vi "人脸识别程序_调用DB匹配_模板匹配.vi"() -> (1 "识别结果":string, 2 "匹配图像":T1(plugin-control))   [LabVIEW 2017]
uses:
  <vilib>/vision/NI_Vision_Development_Module.lvlib
panel:
  out "匹配图像路径":path
  out "Score":sgl
  out "识别成功":bool
  out "添加的路径":path
  out "Number of Matches":i32
  out "Matches (pixel)":T2(array[cluster]) {"Bounding Box"."y" format="%.2f"; "Bounding Box"."x" format="%.2f"; "Score" format="%.2f"; "Scale" format="%.2f"; "Angle" format="%.2f"; "Position"."y" format="%.2f"; "Position"."x" format="%.2f"}
  out "模板图像":T1(plugin-control)
  in  "人脸DB基路径":path=path "D:/机器视觉_短学期/课程项目/人脸图像DB"
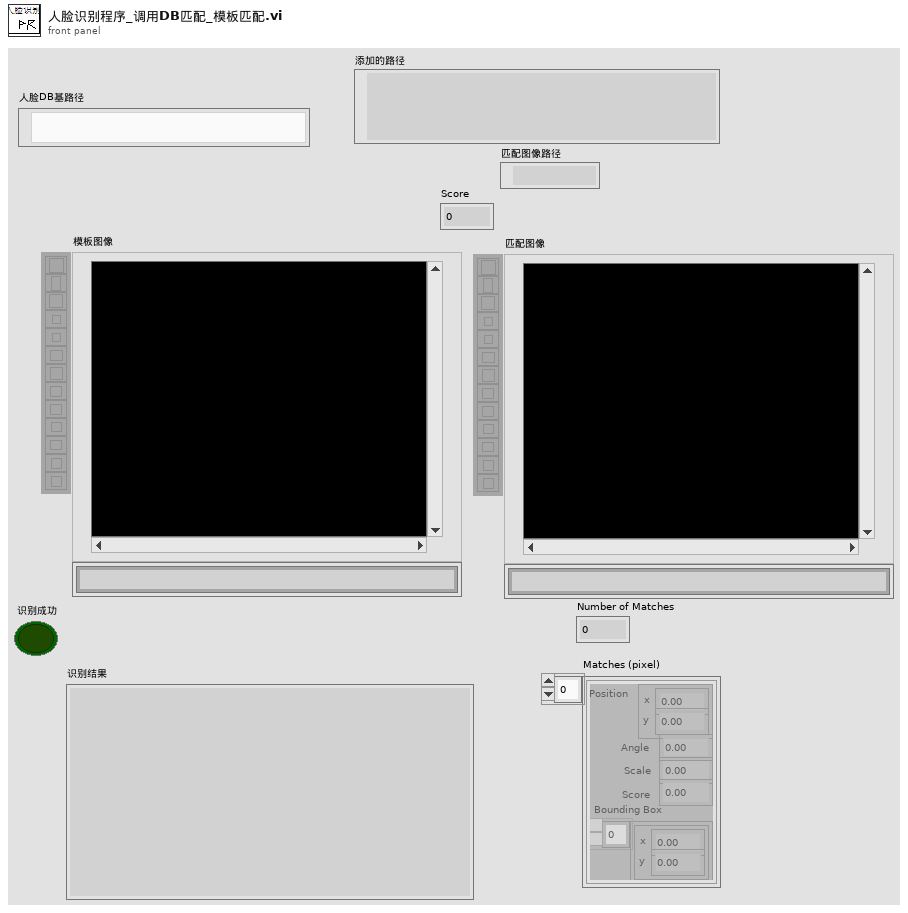
[diagram p1: front panel]
types:
  T1 = typedef "IMAQ Image.ctl" = refnum<image>
  T2 = cluster{"Position":cluster{"x":sgl, "y":sgl}, "Angle":sgl, "Scale":sgl, "Score":sgl, "Bounding Box":cluster{"x":sgl, "y":sgl}[]}[]
  T3 = typedef "Image Type" = u32
  T4 = cluster{"Position":cluster{"x":sgl, "y":sgl}, "Angle":sgl, "Scale":sgl, "Score":sgl, "Bounding Box":cluster{"x":sgl, "y":sgl}[]}
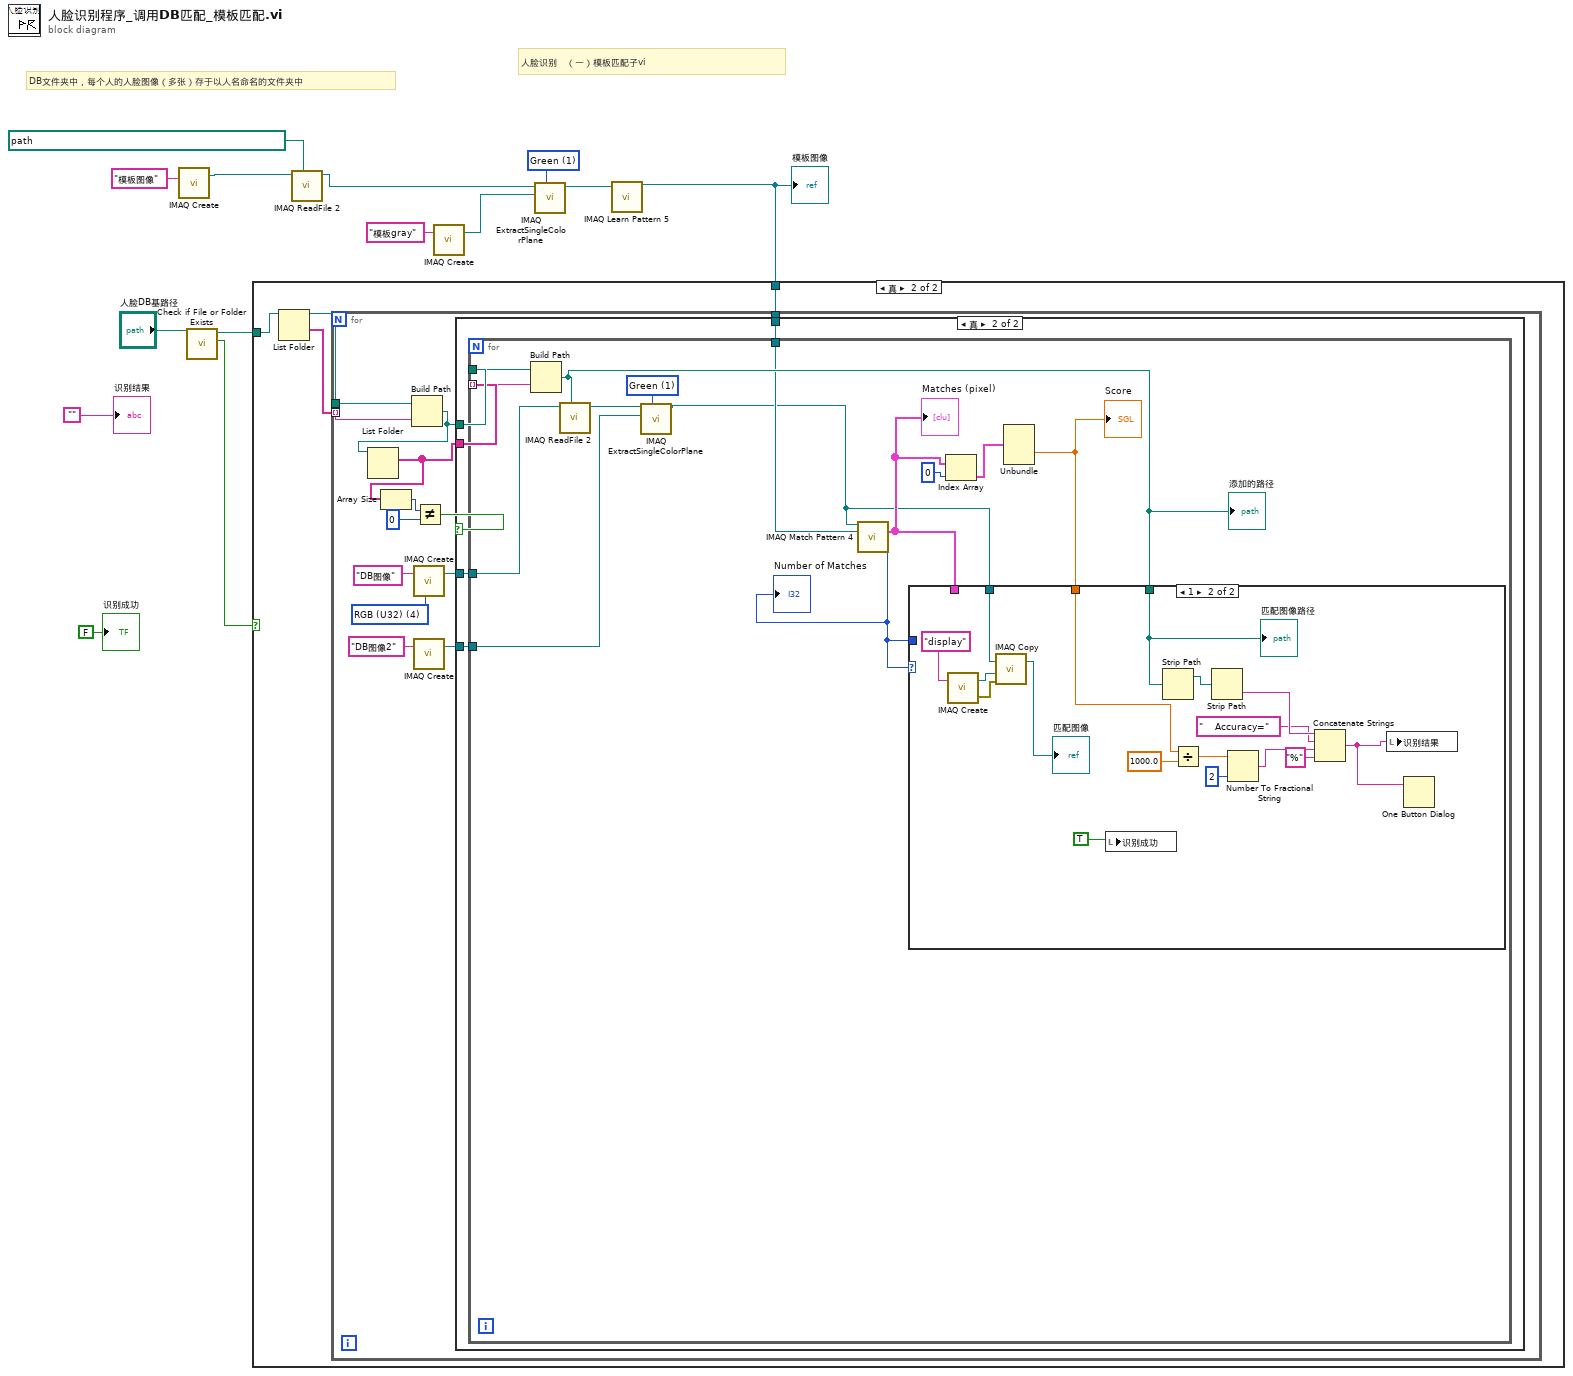
[diagram p0: block diagram]
diagram:
  w11 = 1 items=["Red", "Green", "Blue", "Hue", "Saturation", "Luminance", "Value", "Intensity"] ("Color Plane")
  # "人脸识别   （一）模板匹配子vi"
  # "DB文件夹中，每个人的人脸图像（多张）存于以人名命名的文件夹中"
  n1 = call "IMAQ Create"("Image Name"="模板图像") -> ("New Image"=w4:T1)  [unwired: 4 in, 1 out]
  n2 = call <vilib>:"Check if File or Folder Exists.vi"("path"="人脸DB基路径") -> ("file or folder exists?"=w13:bool, "dup path"=w12:path)  [unwired: 8 in, 1 out]
  n3 = call "IMAQ ReadFile 2"("File Path"=path "D:/机器视觉_短学期/课程项目/人脸图像DB/5.jpg", "Image"=w4) -> ("Image Out"=w1:T1)  [unwired: 5 in, 4 out]
  n4 = call "IMAQ Create"("Image Name"="模板gray") -> ("New Image"=w6:T1)  [unwired: 4 in, 1 out]
  n5 = call "IMAQ ExtractSingleColorPlane"("Color Plane"=w11, "Image Dst"=w6, "Image Src"=w1) -> ("Image Dst Out"=w10:T1)  [unwired: 7 in, 1 out]
  n6 = call "IMAQ Learn Pattern 5"("Image"=w10) -> ("Template Image Out"=w9:T1)  [unwired: 12 in, 2 out]
  "模板图像" <- w9
  n7 = case shown="真" w13 {
    tunnel: w12 -> [_ w18]
    tunnel: w9 -> [_ w15]
    frame False {
    }
    frame True {
      n8 = List Folder(path=w18) -> (path out=w17:path, folder names=w16:string[])  [unwired: 3 in, 2 out]
      n9 = for {
        tunnel: w16 -> [w31] mode=indexing
        tunnel: w17 -> [w25]
        tunnel: w15 -> [w19]
        w23 = T3 4 items=["Grayscale (U8)", "Grayscale (I16)", "Grayscale (SGL)", "Complex (CSG)", "RGB (U32)", "HSL (U32)", "RGB (U64)", "Grayscale (U16)"] ("Image Type")
        n10 = Build Path(base path=w25, name or relative path=w31) -> (appended path=w27:path)
        n11 = List Folder(path=w27) -> (filenames=w26:string[])  [unwired: 3 in, 3 out]
        n12 = Array Size(array=w26) -> (size(s)=w30:i32)
        n13 = call "IMAQ Create"("Image Name"="DB图像", "Image Type"=w23) -> ("New Image"=w22:T1)  [unwired: 3 in, 1 out]
        n14 = call "IMAQ Create"("Image Name"="DB图像2") -> ("New Image"=w20:T1)  [unwired: 4 in, 1 out]
        n15 = Not Equal?(x=w30, y=0) -> (x != y?=w28:bool)
        n16 = case shown="真" w28 {
          tunnel: w27 -> [_ w36]
          tunnel: w26 -> [_ w35]
          tunnel: w22 -> [_ w34]
          tunnel: w20 -> [_ w33]
          tunnel: w19 -> [_ w32]
          frame False {
          }
          frame True {
            n17 = for {
              tunnel: w36 -> [w50]
              tunnel: w35 -> [w49] mode=indexing
              tunnel: w34 -> [w48]
              tunnel: w33 -> [w46]
              tunnel: w32 -> [w41]
              w45 = 1 items=["Red", "Green", "Blue", "Hue", "Saturation", "Luminance", "Value", "Intensity"] ("Color Plane")
              n18 = Build Path(base path=w50, name or relative path=w49) -> (appended path=w42:path)
              "添加的路径" <- w42
              n19 = call "IMAQ ReadFile 2"("File Path"=w42, "Image"=w48) -> ("Image Out"=w47:T1)  [unwired: 5 in, 4 out]
              n20 = call "IMAQ ExtractSingleColorPlane"("Color Plane"=w45, "Image Dst"=w46, "Image Src"=w47) -> ("Image Dst Out"=w37:T1)  [unwired: 7 in, 1 out]
              n21 = call "IMAQ Match Pattern 4"("Image"=w37, "Template Image"=w41) -> ("Matches (pixel)"=w40:T2, "Number of Matches"=w39:i32)  [unwired: 9 in, 3 out]
              "Matches (pixel)" <- w40
              "Number of Matches" <- w39
              n22 = Index Array(array=w40, index=0 ("索引")) -> (element=w43:T4)
              n23 = Unbundle(w43) -> ("Score"=w38:sgl)  [unwired: 4 out]
              "Score" <- w38
              n24 = case shown="1" w39 {
                tunnel: w42 -> [_ w59]
                tunnel: w39 -> [_ _]
                tunnel: w40 -> [_ _]
                tunnel: w38 -> [_ w57]
                tunnel: w37 -> [_ w56]
                frame 0, Default {
                }
                frame 1 {
                  n25 = call "IMAQ Create"("Image Name"="display") -> ("New Image"=w55:T1, "error out"=w54:errorcluster)  [unwired: 4 in]
                  n26 = call "IMAQ Copy"("error in (no error)"=w54, "Image Dst"=w55, "Image Src"=w56) -> ("Image Dst Out"=→"匹配图像":T1)  [unwired: 3 in, 1 out]
                  n27 = local write "识别成功"(TRUE) -> ()
                  n28 = Strip Path(path=w59) -> (stripped path=w64:path)  [unwired: 1 out]
                  n29 = Divide(x=w57, y=sgl 1000.0) -> (x/y=w65:sgl)
                  n30 = Strip Path(path=w64) -> (name=w66:string)  [unwired: 1 out]
                  n31 = Number To Fractional String(number=w65, precision (6)=i16 2 ("精度(6)")) -> (F-format string=w67:string)  [unwired: 2 in]
                  n32 = Concatenate Strings(w66, "    Accuracy=" ("字符串"), w67, "%" ("字符串")) -> (w51:string)
                  n33 = local write "识别结果"(w51) -> ()
                  n34 = One Button Dialog(message=w51) -> ()  [unwired: 1 in, 1 out]
                  "匹配图像路径" <- w59
                }
              }
            }
          }
        }
      }
    }
  }
  "识别结果" <- ""
  "识别成功" <- FALSE ("识别成功")
